vi "InsituInit.vi"(7 "Current(A)":dbl, 8 "error in (no error)":errorcluster, 11 "Instruments in":refnum<class "Instruments.lvclass">) -> (0 "error out":errorcluster, 3 "Instruments out":refnum<class "Instruments.lvclass">)   [LabVIEW 2012, in "Instruments.lvclass"]
uses:
  Instruments.lvclass
  Controls/SpectrometerOphirSelector.ctl
  Instruments.lvclass/Instruments.ctl
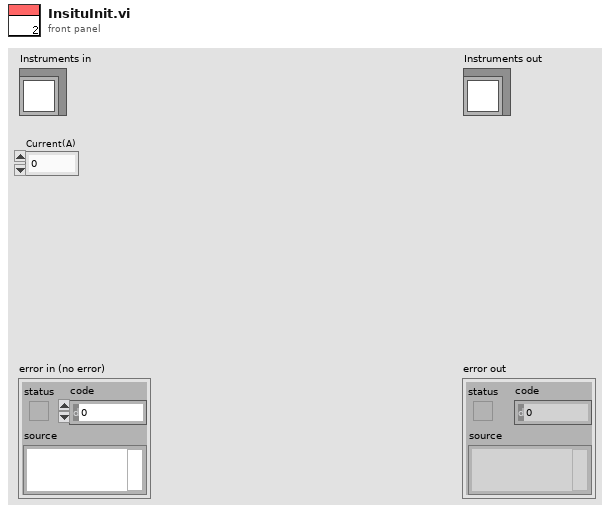
[diagram p1: front panel]
types:
  T1 = typedef "SpectrometerOphirSelector.ctl" = enum16{"Get Background", "Measure", "Measure50", "Raw"}
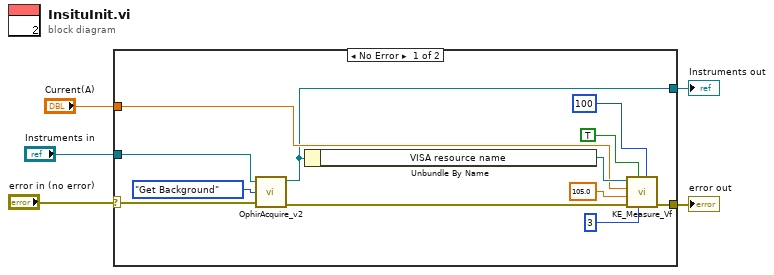
[diagram p0: block diagram]
diagram:
  n1 = case shown="No Error" "error in (no error)" {
    selector: "error in (no error)" -> [w9 w19]
    tunnel: [w8 w19] -> w4
    tunnel: [w6 w18] -> w2
    tunnel: "Instruments in" -> [w12 w18]
    tunnel: "Current(A)" -> [w7 _]
    frame No Error {
      n2 = call-dynamic "OphirAcquire_v2.vi"("Instruments in"=w12, "Type"=SpectrometerOphirSelector."Get Background", "error in (no error)"=w9) -> ("Instruments out"=w6:refnum<class "Instruments.lvclass">, "error out"=w10:errorcluster)  [unwired: 2 out]
      n3 = Unbundle By Name(w6) -> ("VISA resource name"=w11:refnum<visa-resource-name>)
      n4 = call "KE_Measure_Vf.vi"("Settle Delay"=u32 100, "Samples"=3, "Keep On"=TRUE, "error in (no error)"=w10, "Compliance"=105.0, "Current(A)"=w7, "KE_In"=w11) -> ("error out"=w8:errorcluster)  [unwired: 2 in, 2 out]
    }
    frame Error {
    }
  }
  "error out" <- w4
  "Instruments out" <- w2
